vi "Add Timestamp.vi"(1 "data in":T1={"X"=0, "Y"=0, "Z"=0, "flame"=TRUE, "magnet"=TRUE, "obstacle"=FALSE, "sound"=[]}, 2 "current time":timestamp) -> (0 "data out":waveform(i8)[](array[waveform]))   [LabVIEW 2015]
uses:
  Sensors Data.ctl
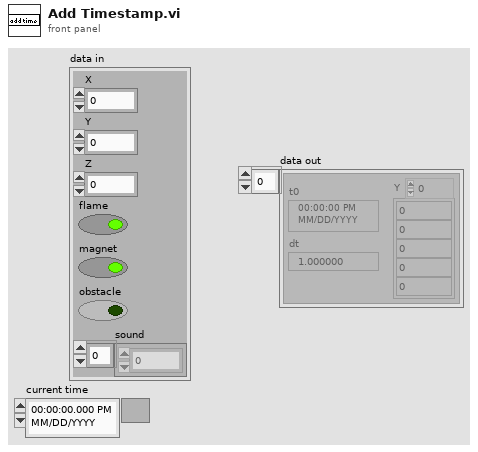
[diagram p1: front panel]
types:
  T1 = typedef "Sensors Data.ctl" = cluster{"X":i8, "Y":i8, "Z":i8, "flame":bool, "magnet":bool, "obstacle":bool, "sound":sgl[]}
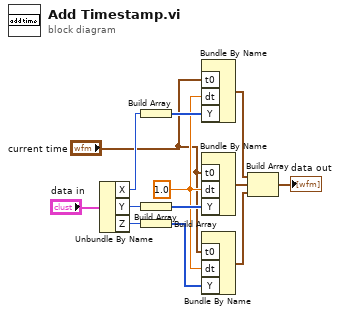
[diagram p0: block diagram]
diagram:
  w3 = 1.0 ("dt")
  n1 = Unbundle By Name("data in") -> ("X"=w9:i8, "Y"=w8:i8, "Z"=w7:i8)
  n2 = Build Array(w9) -> (w12:i8[])
  n3 = Build Array(w8) -> (w11:i8[])
  n4 = Build Array(w7) -> (w10:i8[])
  n5 = Bundle By Name("t0"="current time", "dt"=w3, "Y"=w12) -> (w5:waveform(i8))  [unwired: 1 in]
  n6 = Bundle By Name("t0"="current time", "dt"=w3, "Y"=w11) -> (w4:waveform(i8))  [unwired: 1 in]
  n7 = Bundle By Name("t0"="current time", "dt"=w3, "Y"=w10) -> (w6:waveform(i8))  [unwired: 1 in]
  n8 = Build Array(w5, w4, w6) -> (→"data out":waveform(i8)[])
